vi "tsapp_transmit_lin_sync.vi"(8 "错误输入（无错误）":errorcluster, 9 "ATimeoutMS":i32, 10 "LIN_Transmit":T1 {"Channel" items=["CHN1", "CHN2", "CHN3", "CHN4", "CHN5", "CHN6", "CHN7", "CHN8", "CHN9", "CHN10", "CHN11", "CHN12", "CHN13", "CHN14", "CHN15", "CHN16", "CHN17", "CHN18", "CHN19", "CHN20", "CHN21", "CHN22", "CHN23", "CHN24", "CHN25", "CHN26", "CHN27", "CHN28", "CHN29", "CHN30", "CHN31", "CHN32"]; "ID" format="%.0x"; "DLC" format="%.0x"; "Set_node_funtiontype" items=["MasterNode", "SlaveNode", "MonitorNote"]}, 11 "路径输入":path) -> (0 "错误输出":errorcluster, 2 "return":i32, 3 "路径输出":path)   [LabVIEW 2014]
doc: "Function Introduction :\nSynchronize transmission of LIN messages, current execution is blocked until the frame is sent or timed out\nCall location :\ninput parameter :\nALIN: Pointer to lin data structure\nATimeoutMS: timeout (milliseconds)\nReturn value :\n==0: Execution successful\nOther values: Query error code"
uses:
  Typedef/TLibLIN.ctl
  Typedef/TSLIN_Transmit.ctl
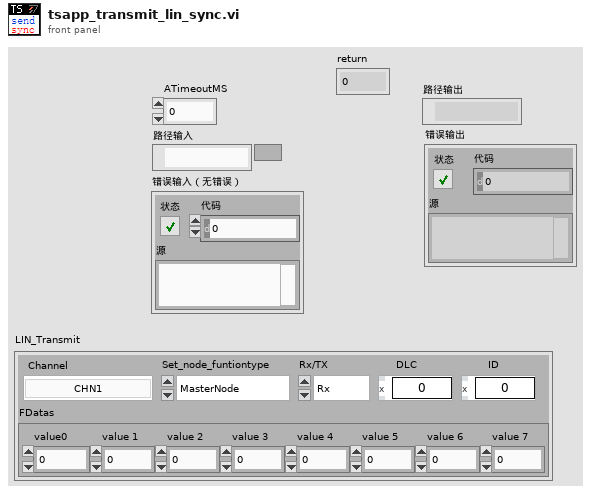
[diagram p1: front panel]
types:
  T1 = typedef "TSLIN_Transmit.ctl" = cluster{"Channel":i32, "Rx/TX":enum16{"Rx", "Tx"}, "Set_node_funtiontype":i32, "DLC":u32, "ID":u32, "FDatas":cluster{"value0":u8, "value 1":u8, "value 2":u8, "value 3":u8, "value 4":u8, "value 5":u8, "value 6":u8, "value 7":u8}}
  T2 = typedef "TLibLIN.ctl" = cluster{"Ch":u8, "Code":u8, "Properties":u8, "FDLC":u8, "ID":u8, "Checksum":u8, "FStaus":u8, "FTimeUS":u64, "FDatas":cluster{"value0":u8, "value 1":u8, "value 2":u8, "value 3":u8, "value 4":u8, "value 5":u8, "value 6":u8, "value 7":u8}}
  T3 = cluster{"value0":u8, "value 1":u8, "value 2":u8, "value 3":u8, "value 4":u8, "value 5":u8, "value 6":u8, "value 7":u8}
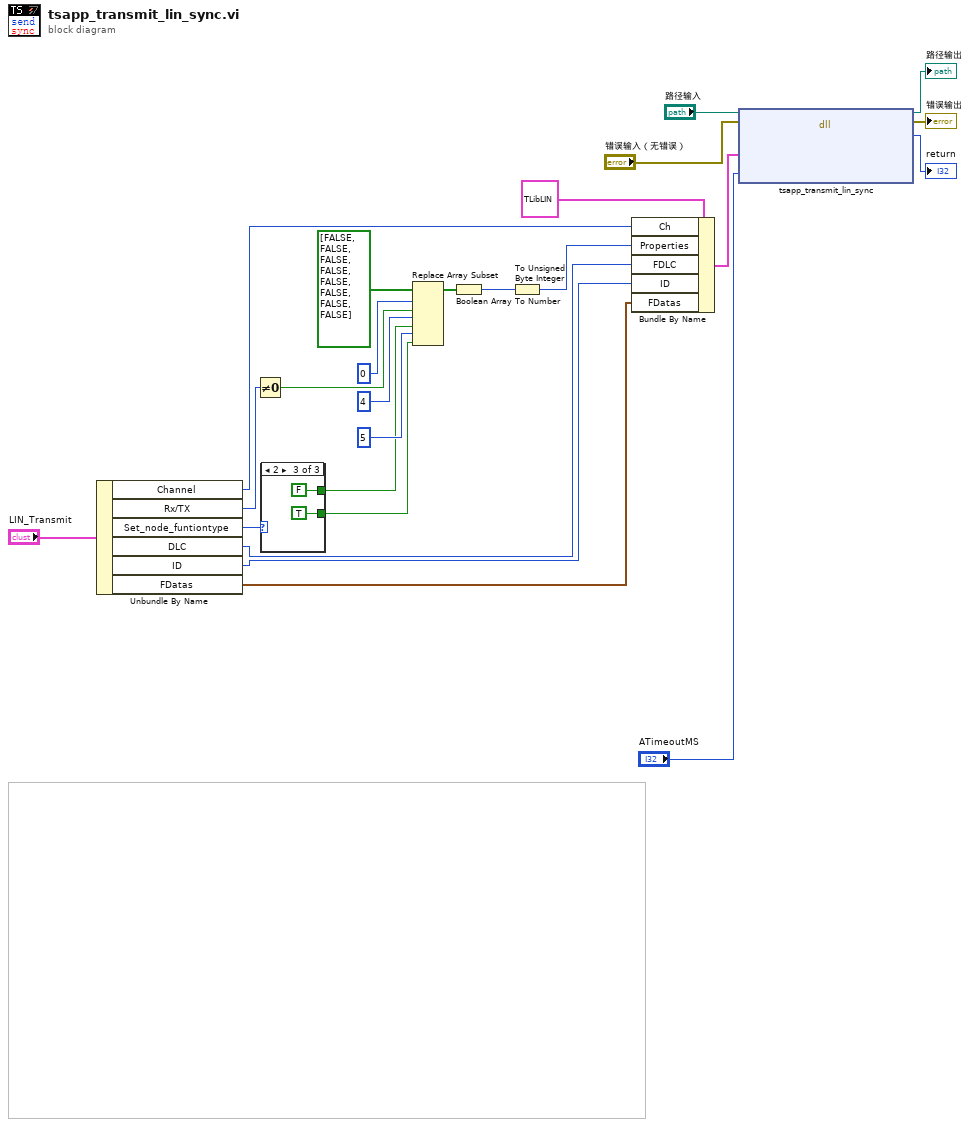
[diagram p0: block diagram]
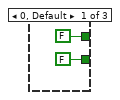
[diagram p2: hidden frame]
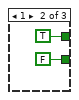
[diagram p3: hidden frame]
diagram:
  n1 = Unbundle By Name("LIN_Transmit") -> ("Channel"=w19:i32, "Rx/TX"=w15:enum16{"Rx", "Tx"}, "Set_node_funtiontype"=w11:i32, "DLC"=w17:u32, "ID"=w18:u32, "FDatas"=w1:T3)
  n2 = Not Equal To 0?(x=w15) -> (x != 0?=w14:bool)
  n3 = case shown="2" w11 {
    tunnel: [FALSE TRUE FALSE] -> w10
    tunnel: [FALSE FALSE TRUE] -> w9
    frame 0, Default {
    }
    frame 1 {
    }
    frame 2 {
    }
  }
  n4 = Replace Array Subset(array=bool[] [FALSE, FALSE, FALSE, FALSE, FALSE, FALSE, FALSE, FALSE], new element #1=w14, index #1=0 ("索引"), new element #2=w10, index #2=4 ("索引"), new element #3=w9, index #3=5 ("索引")) -> (w23:bool[])
  n5 = Boolean Array To Number(Boolean array=w23) -> (number=w22:u32)
  n6 = To Unsigned Byte Integer(number=w22) -> (unsigned 8bit integer=w21:u8)
  n7 = Bundle By Name(cluster=T2 {"Ch"=0, "Code"=0, "Properties"=0, "FDLC"=0, "ID"=0, "Checksum"=0, "FStaus"=0, "FTimeUS"=0, "FDatas"={"value0"=0, "value 1"=0, "value 2"=0, "value 3"=0, "value 4"=0, "value 5"=0, "value 6"=0, "value 7"=0}} ("TLIBLIN"), "Ch"=w19, "Properties"=w21, "FDLC"=w17, "ID"=w18, "FDatas"=w1) -> (w8:T2)
  n8 = dll-call lib="D:/Program Files (x86)/TOSUN/TSMaster/Data/SDK/lib/x86/TSMaster.dll" fn="tsapp_transmit_lin_sync"(path in="路径输入", error in="错误输入（无错误）", "ALIN"=w8, "ATimeoutMS"="ATimeoutMS") -> (path out=→"路径输出":path, error out=→"错误输出":errorcluster, "返回类型"=→"return":i32)  [unwired: 3 in]
